vi "DEV - check cluster matches database cols.vi"(8 "Error In":errorcluster, 11 "Generic Cluster Reference":refnum<vi>) -> (0 "Error Out":errorcluster, 3 "Cluster matches DB?":bool[](array[boolean]))   [LabVIEW 2018, in "Database.lvlib"]
uses:
  Database.lvlib
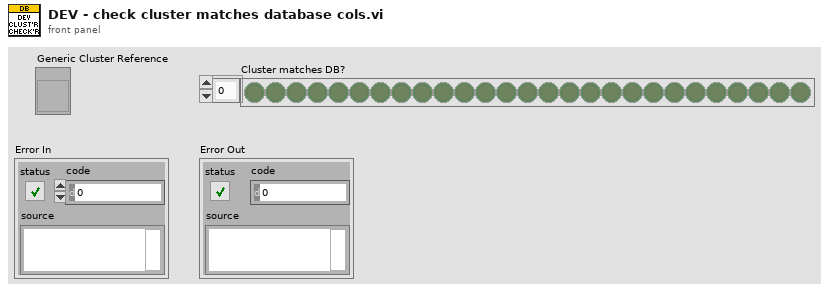
[diagram p1: front panel]
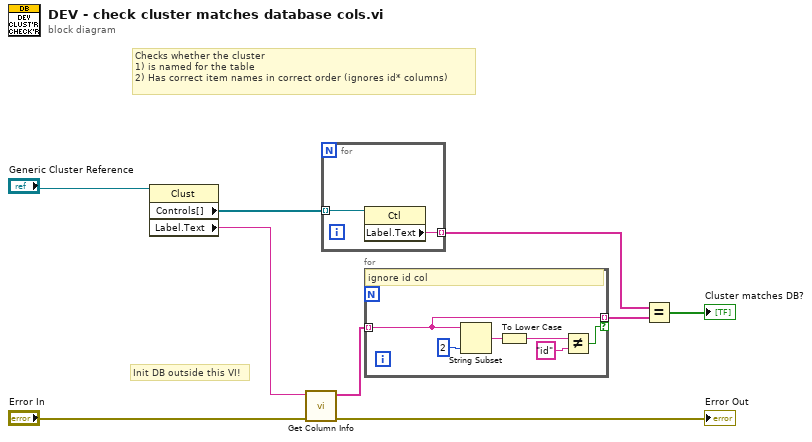
[diagram p0: block diagram]
diagram:
  # "Init DB outside this VI!"
  # "Checks whether the cluster \n1) is named for the table\n2) Has correct item names in correct order (ignores id* columns)"
  n1 = property class="Clust"(reference="Generic Cluster Reference") -> ("Controls[]"=w2:refnum<vi>[], "Label.Text"=w3:string)  [unwired: 1 in, 2 out]
  n2 = call "Get Column Info.vi"("Error In"="Error In", "Table"=w3) -> ("Error Out"=→"Error Out":errorcluster, "Column Names"=w6:string[])  [unwired: 7 in, 1 out]
  n3 = for {
    tunnel: w2 -> [w11] mode=indexing
    tunnel: [w10] -> w4 mode=indexing
    n4 = property class="Ctl"(reference=w11) -> ("Label.Text"=w10:string)  [unwired: 1 in, 2 out]
  }
  n5 = for {
    tunnel: w6 -> [w13] mode=indexing
    tunnel: [w13] -> w7 mode=indexing if=w12
    # "ignore id col"
    n6 = String Subset(string=w13, length (rest)=2 ("length (rest)")) -> (substring=w14:string)  [unwired: 1 in]
    n7 = To Lower Case(string=w14) -> (all lower case string=w15:string)
    n8 = Not Equal?(x=w15, y="id") -> (x != y?=w12:bool)
  }
  n9 = Equal?(x=w4, y=w7) -> (x = y?=→"Cluster matches DB?":bool[])
